vi "calculateFFT.vi"(8 "ErrorIn":errorcluster, 11 "AccelerationDataIn":waveform(dbl)[](array[waveform])) -> (0 "ErrorOut":errorcluster, 2 "AccelerationDataFrames":T1, 3 "AccelerationDataOut":waveform(dbl)[](array[waveform]))   [LabVIEW 2019]
uses:
  AccelerationDataFrames.ctl
  <vilib>/measure/madcrms.llb/Basic Averaged DC-RMS for 1 Chan.vi
  <vilib>/measure/maspectr.llb/FFT Spectrum (Real-Im) for 1 Chan.vi
  <vilib>/measure/NI_MAPro.lvlib
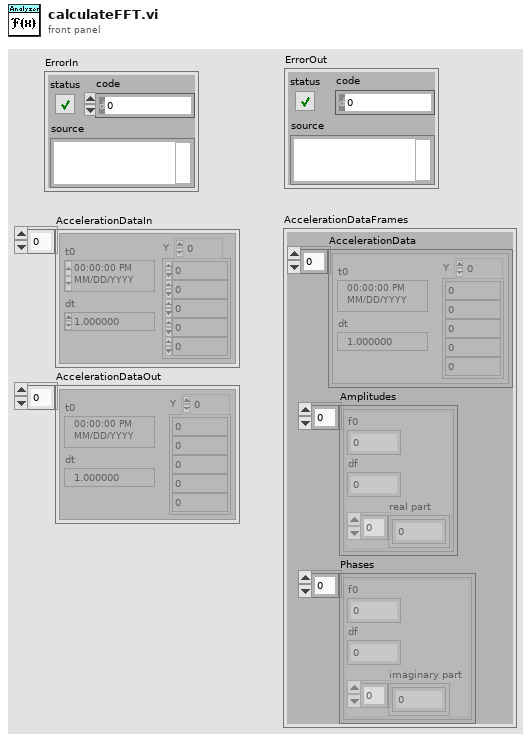
[diagram p1: front panel]
types:
  T1 = typedef "AccelerationDataFrames.ctl" = cluster{"AccelerationData":waveform(dbl)[], "Amplitudes":cluster{"f0":dbl, "df":dbl, "real part":dbl[]}[], "Phases":cluster{"f0":dbl, "df":dbl, "imaginary part":dbl[]}[]}
  T2 = cluster{"averaging mode":enum16{"No averaging", "Vector averaging", "RMS averaging", "Peak hold"}, "weighting mode":enum16{"Linear", "Exponential"}, "number of averages":u32}
  T3 = enum16{"Rectangular (none)", "Hanning", "Low side lobe"}
  T4 = cluster{"f0":dbl, "df":dbl, "imaginary part":dbl[]}
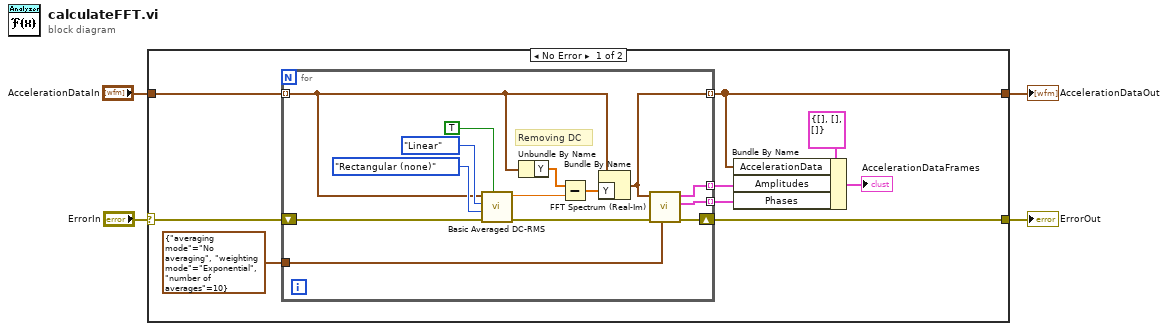
[diagram p0: block diagram]
diagram:
  n1 = case shown="No Error" "ErrorIn" {
    selector: "ErrorIn" -> [w7 w29]
    tunnel: [w13 w29] -> w4
    tunnel: "AccelerationDataIn" -> [w6 w28]
    tunnel: [w5 w28] -> w1
    frame No Error {
      n2 = for {
        shift-right: [w27] -> w13
        shift-left: w7 -> [w23]
        tunnel: T2 {"averaging mode"=enum."No averaging", "weighting mode"=enum."Exponential", "number of averages"=10} ("averaging parameters") -> [w26]
        tunnel: [w25] -> w10 mode=indexing
        tunnel: [w24] -> w9 mode=indexing
        tunnel: w6 -> [w16] mode=indexing
        tunnel: [w14] -> w5 mode=indexing
        # "Removing DC"
        n3 = call-poly <vilib>:"Basic Averaged DC-RMS.vi"("reset"=TRUE, "error in (no error)"=w23, "window"=T3."Rectangular (none)", "averaging type"=enum16{"Linear", "Exponential"}."Linear", "signal in"=w16) -> ("error out"=w17:errorcluster, "DC value"=w19:dbl)  [unwired: 3 in, 2 out]
        n4 = Unbundle By Name(w16) -> ("Y"=w18:dbl[])
        n5 = Subtract(x=w18, y=w19) -> (x-y=w15:dbl[])
        n6 = Bundle By Name(cluster=w16, "Y"=w15) -> (w14:waveform(dbl))
        n7 = call-poly <vilib>:"FFT Spectrum (Real-Im).vi"("averaging parameters"=w26, "error in (no error)"=w17, "time signal"=w14) -> ("error out"=w27:errorcluster, "imaginary part"=w24:T4, "real part"=w25:cluster{"f0":dbl, "df":dbl, "real part":dbl[]})  [unwired: 4 in, 2 out]
      }
      n8 = Bundle By Name(cluster=T1 {"AccelerationData"=[], "Amplitudes"=[], "Phases"=[]} ("AccelerationDataFrames"), "AccelerationData"=w5, "Amplitudes"=w10, "Phases"=w9) -> (→"AccelerationDataFrames":T1)
    }
    frame Error {
    }
  }
  "ErrorOut" <- w4
  "AccelerationDataOut" <- w1
